vi "DisconnectBase.vi"(8 "error in (no error)":errorcluster, 11 "National Instruments USB-8473 Adapter Class in":refnum<class "National Instruments USB-8473 Adapter Class.lvclass">) -> (0 "error out":errorcluster, 3 "National Instruments USB-8473 Adapter Class out":refnum<class "National Instruments USB-8473 Adapter Class.lvclass">)   [LabVIEW 2011, in "National Instruments USB-8473 Adapter Class.lvclass"]
uses:
  National Instruments USB-8473 Adapter Class.lvclass
  Generic CAN Adapter/GenericCanAdapterClass.lvclass
  National Instruments USB-8473 Adapter Class.lvclass/National Instruments USB-8473 Adapter Class.ctl
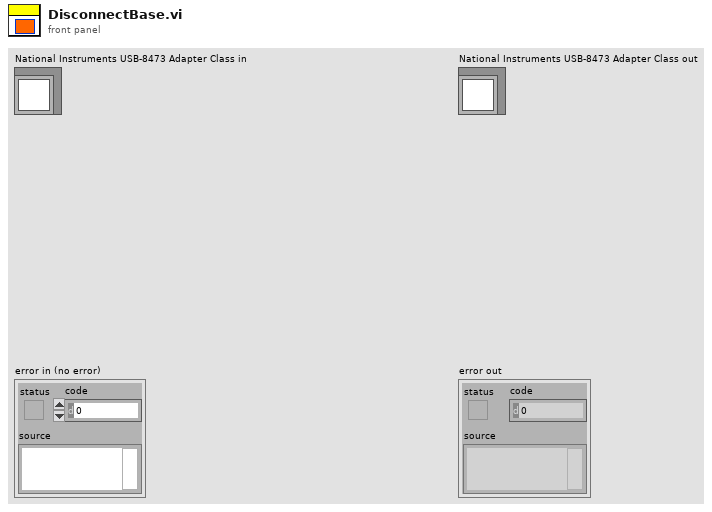
[diagram p1: front panel]
types:
  T1 = typedef "xobjhandle.ctl" = u32
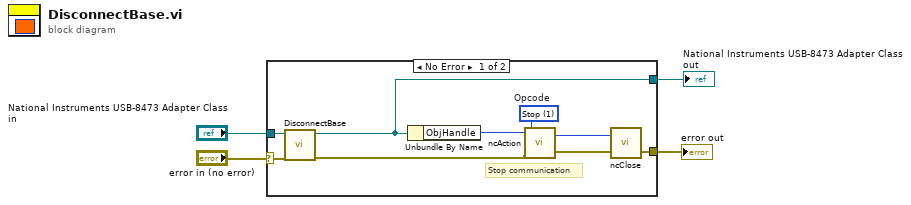
[diagram p0: block diagram]
diagram:
  n1 = case shown="No Error" "error in (no error)" {
    selector: "error in (no error)" -> [w5 w14]
    tunnel: "National Instruments USB-8473 Adapter Class in" -> [w13 w15]
    tunnel: [w9 w15] -> w3
    tunnel: [w6 w14] -> w2
    frame No Error {
      w10 = u32 1 items=["Start", "Stop", "Reset", "Output on RTSI line"]  # Opcode
      # "Stop communication"
      n2 = call-parent "DisconnectBase.vi"("error in (no error)"=w5, "GenericCanAdapterClass in"=w13) -> ("error out"=w7:errorcluster, "GenericCanAdapterClass out"=w9:refnum<class "National Instruments USB-8473 Adapter Class.lvclass">)  [unwired: 8 in]
      n3 = Unbundle By Name(w9) -> ("ObjHandle"=w8:T1)
      n4 = call <vilib>:"ncAction.vi"("Error in"=w7, "Opcode"=w10, "ObjHandle in"=w8) -> ("Error out"=w12:errorcluster, "ObjHandle out"=w11:T1)  [unwired: 1 in]
      n5 = call <vilib>:"ncClose.vi"("Error in"=w12, "ObjHandle in"=w11) -> ("Error out"=w6:errorcluster)  [unwired: 1 in]
    }
    frame Error {
    }
  }
  "error out" <- w2
  "National Instruments USB-8473 Adapter Class out" <- w3
